vi "WAM_UserInfo_Prompt.vi"(0 "Enable":bool=TRUE, 11 "error in (no error)":errorcluster) -> (1 "Bar Code":string, 2 "BarCodeInfo":string, 3 "BC_MSN":string, 4 "cancelled?(t)":bool, 15 "error out":errorcluster)   [LabVIEW 2018]
panel:
  out "Company":string
  out "BC_ESN":string
  out "LotID":string
  out "Revision":string
  out "Rage PN":string
  out "match substring":string
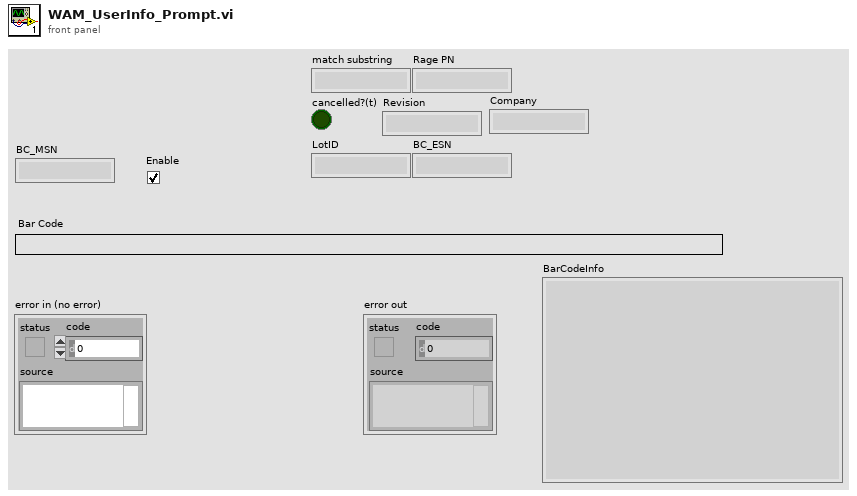
[diagram p1: front panel]
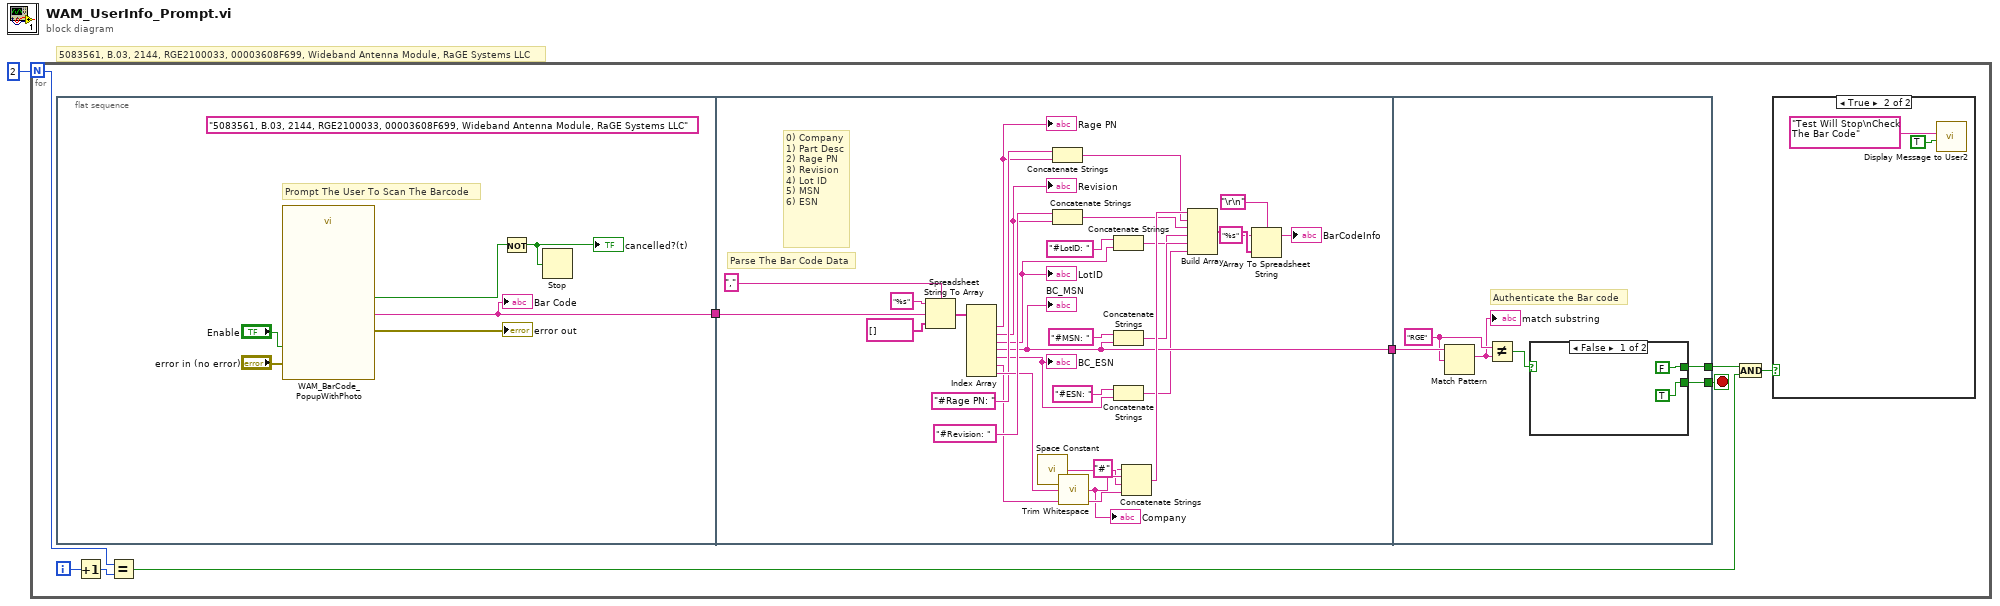
[diagram p0: block diagram]
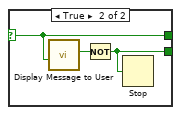
[diagram p3: hidden frame]
diagram:
  # "5083561, B.03, 2144, RGE2100033, 00003608F699, Wideband Antenna Module, RaGE Systems LLC"
  n1 = for {
    N: 2 -> [w7]
    i -> [w8]
    stop <- w5 stop-if-true
    n2 = flat-sequence {
      tunnel: [w13] -> w10
      tunnel: w10 -> [w48]
      tunnel: [w30] -> w9
      tunnel: w9 -> [w54]
      tunnel: [w51] -> w5
      tunnel: [w49] -> w2
      frame #0 {
        (unwired) "5083561, B.03, 2144, RGE2100033, 00003608F699, Wideband Antenna Module, RaGE Systems LLC" ("Bar Code")
        # "Prompt The User To Scan The Barcode"
        n3 = call "WAM_BarCode_PopupWithPhoto.vi"("Enable"="Enable", "error in (no error)"="error in (no error)") -> ("Bar Code"=w13:string, "OK"=w16:bool, "error out"=→"error out":errorcluster)  [unwired: 15 in]
        "Bar Code" <- w13
        n4 = Not(x=w16) -> (.not. x?=w14:bool)
        "cancelled?(t)" <- w14
        n5 = Stop(stop? (T)=w14) -> ()
      }
      frame #1 {
        # "0) Company\n1) Part Desc\n2) Rage PN\n3) Revision \n4) Lot ID\n5) MSN\n6) ESN"
        # "Parse The Bar Code Data"
        n6 = Spreadsheet String To Array(delimiter (Tab)=",", format string="%s", spreadsheet string=w48, array type (2D Dbl)=string[] []) -> (array=w44:string[])
        n7 = Index Array(array=w44) -> (element #1=w35:string, element #2=w33:string, element #3=w32:string, element #4=w30:string, element #5=w28:string, element #6=w22:string, element #7=w39:string)  [unwired: 7 in]
        "BC_MSN" <- w30
        "Rage PN" <- w35
        "Revision" <- w33
        "LotID" <- w32
        "BC_ESN" <- w28
        n8 = call <vilib>:"Space Constant.vi"() -> ("String"=w20:string)
        n9 = Concatenate Strings("#Rage PN: ", w35) -> (w36:string)
        n10 = Concatenate Strings("#Revision: ", w33) -> (w34:string)
        n11 = call <vilib>:"Trim Whitespace.vi"("string"=w39) -> ("trimmed string"=w21:string)  [unwired: 1 in]
        "Company" <- w21
        n12 = Concatenate Strings("#LotID: ", w32) -> (w27:string)
        n13 = Concatenate Strings("#MSN: ", w30) -> (w31:string)
        n14 = Concatenate Strings("#ESN: ", w28) -> (w29:string)
        n15 = Concatenate Strings("#" ("string"), w21, w20, w22) -> (w38:string)
        n16 = Build Array(w38, w36, w34, w27, w31, w29) -> (w25:string[])
        n17 = Array To Spreadsheet String(delimiter (Tab)="\r\n", array=w25, 3:"%s" ("format string")) -> (spreadsheet string=→"BarCodeInfo":string)
      }
      frame #2 {
        w53 = "RGE" ("regular expression")
        # "Authenticate the Bar code"
        n18 = Match Pattern(string=w54, regular expression=w53) -> (match substring=w52:string)  [unwired: 1 in, 3 out]
        "match substring" <- w52
        n19 = Not Equal?(x=w53, y=w52) -> (x != y?=w50:bool)
        n20 = case shown="False" w50 {
          selector: w50 -> [_ w57]
          tunnel: [TRUE w58] -> w51
          tunnel: [FALSE w57] -> w49
          frame False {
          }
          frame True {
            n21 = call "Display Message to User"("Enable"=w57) -> ("OK"=w59:bool)  [unwired: 9 in, 1 out]
            n22 = Not(x=w59) -> (.not. x?=w58:bool)
            n23 = Stop(stop? (T)=w58) -> ()
          }
        }
      }
    }
    n24 = Increment(x=w8) -> (x+1=w6:i32)
    n25 = Equal?(x=w7, y=w6) -> (x = y?=w3:bool)
    n26 = And(x=w2, y=w3) -> (x .and. y?=w4:bool)
    n27 = case shown="True" w4 {
      frame False {
      }
      frame True {
        n28 = call "Display Message to User2"("Enable"=TRUE, "Message"="Test Will Stop\nCheck The Bar Code") -> ()  [unwired: 8 in, 2 out]
      }
    }
  }
